vi "checkTrigger.vi"(6 "Trigger.Mode::1":T1, 9 "Trigger.DigitalSource::1":refnum<vi>, 10 "Trigger.AnalogSource::1":refnum<vi>, 11 "Ring in":refnum<vi>) -> (0 "text":string[](array[string]), 1 "index array":i32[](array[numeric]), 3 "update?":bool)   [LabVIEW 2013]
uses:
  Device Driver/PXIdigitizer/mode_TypDef.ctl
  General-Controler/firstCall_TypDef.ctl
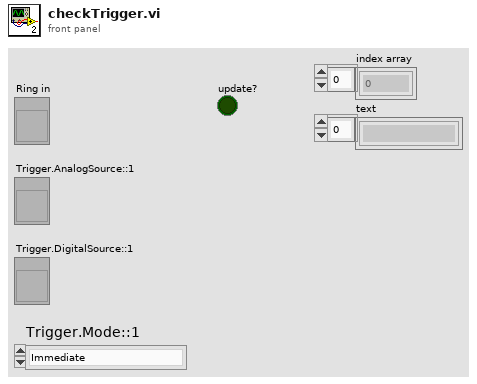
[diagram p1: front panel]
types:
  T1 = typedef "mode_TypDef.ctl" = enum32{"Immediate", "Analog Edge", "Analog Window", "Analog Hysteresis", "Video", "Digital Edge"}
  T2 = typedef "firstCall_TypDef.ctl" = enum16{"reset", "read"}
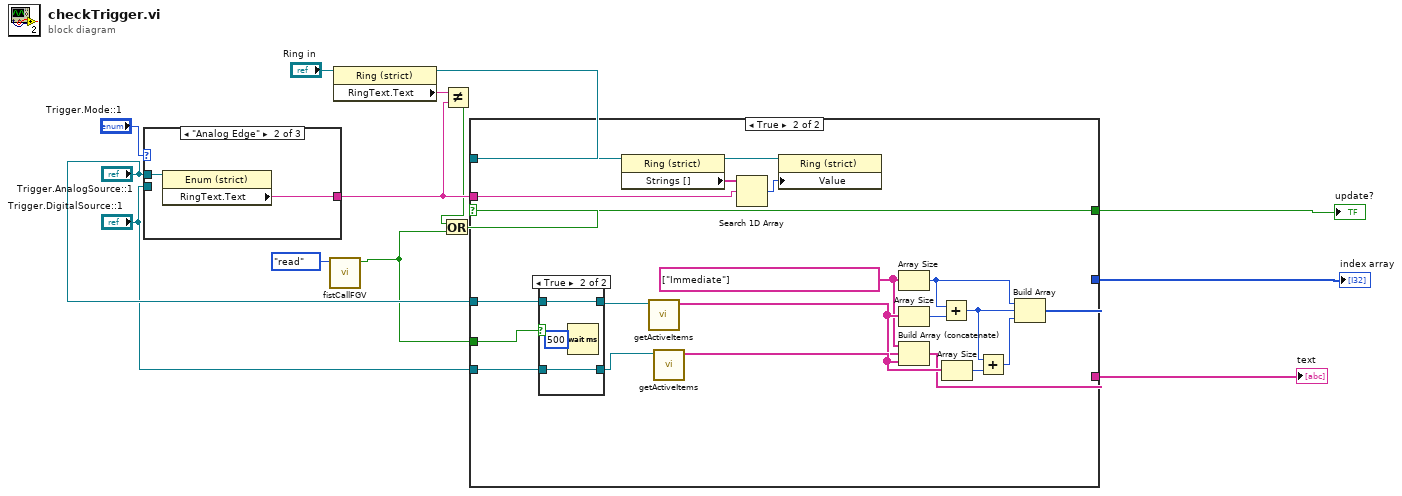
[diagram p0: block diagram]
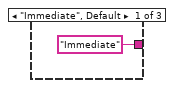
[diagram p4: hidden frame]
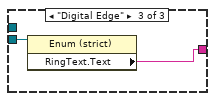
[diagram p5: hidden frame]
diagram:
  n1 = case shown="\"Analog Edge\"" "Trigger.Mode::1" {
    tunnel: ["Immediate" w16 w18] -> w14
    tunnel: "Trigger.AnalogSource::1" -> [_ w17 _]
    tunnel: "Trigger.DigitalSource::1" -> [_ _ w19]
    frame "Immediate", Default {
    }
    frame "Analog Edge" {
      n2 = property class="Enum (strict)"(reference=w17) -> ("RingText.Text"=w16:string)  [unwired: 1 in, 2 out]
    }
    frame "Digital Edge" {
      n3 = property class="Enum (strict)"(reference=w19) -> ("RingText.Text"=w18:string)  [unwired: 1 in, 2 out]
    }
  }
  n4 = call "fistCallFGV.vi"("Function"=firstCall_TypDef."read") -> ("first call out"=w1:bool)  [unwired: 9 in, 1 out]
  n5 = property class="Ring (strict)"(reference="Ring in") -> (reference out=w12:refnum<vi>, "RingText.Text"=w13:string)  [unwired: 1 in, 1 out]
  n6 = Not Equal?(x=w13, y=w14) -> (x != y?=w6:bool)
  n7 = Or(x=w6, y=w1) -> (x .or. y?=w3:bool)
  n8 = case shown="True" w3 {
    selector: w3 -> [w20 w36]
    tunnel: w12 -> [_ w38]
    tunnel: w14 -> [_ w37]
    tunnel: [w20 w36] -> w5
    tunnel: "Trigger.AnalogSource::1" -> [_ w24]
    tunnel: "Trigger.DigitalSource::1" -> [_ w22]
    tunnel: [_ w27] -> w7
    tunnel: [_ w26] -> w4
    tunnel: w1 -> [_ w25]
    frame False {
    }
    frame True {
      w28 = string[] ["Immediate"]
      n9 = case shown="True" w25 {
        tunnel: w24 -> [w43 w46]
        tunnel: [w43 w46] -> w23
        tunnel: w22 -> [w42 w45]
        tunnel: [w42 w45] -> w21
        frame False {
        }
        frame True {
          n10 = Wait (ms)(milliseconds to wait=u32 500) -> ()  [unwired: 1 out]
        }
      }
      n11 = property class="Ring (strict)"(reference=w38) -> (reference out=w41:refnum<vi>, "Strings []"=w40:string[])  [unwired: 1 in, 1 out]
      n12 = call "getActiveItems.vi"("Enum in"=w23) -> ("array w/ subset deleted"=w29:string[])  [unwired: 10 in]
      n13 = call "getActiveItems.vi"("Enum in"=w21) -> ("array w/ subset deleted"=w30:string[])  [unwired: 10 in]
      n14 = Search 1D Array(1D array=w40, element=w37) -> (index of element=w39:i32)  [unwired: 1 in]
      n15 = property class="Ring (strict)"(reference=w41, "Value"=w39) -> ()  [unwired: 1 in, 2 out]
      n16 = Array Size(array=w28) -> (size(s)=w31:i32)
      n17 = Array Size(array=w29) -> (size(s)=w32:i32)
      n18 = Build Array (concatenate)(w28, w29, w30) -> (w26:string[])
      n19 = Add(x=w31, y=w32) -> (x+y=w34:i32)
      n20 = Array Size(array=w30) -> (size(s)=w35:i32)
      n21 = Add(x=w34, y=w35) -> (x+y=w33:i32)
      n22 = Build Array(w31, w34, w33) -> (w27:i32[])
    }
  }
  "update?" <- w5
  "index array" <- w7
  "text" <- w4
